vi "PutSpectralData.vi"(0 "shot":i32, 1 "wavelengths":dbl[](array[numeric]), 2 "Counts":dbl[][](array[numeric]), 3 "time":dbl[](array[numeric]), 4 "Integration Times":i32[](array[numeric]), 5 "LensFiber":string, 6 "Radius 1":dbl, 7 "Radius 2":dbl, 8 "Z 1":dbl=-1.0, 9 "Z 2":dbl=1.0, 10 "Angle 1":dbl=157.5, 11 "Angle 2":dbl=157.5, 12 "Comments":string, 13 "backup_directory":path) -> ()   [LabVIEW 2011]
panel:
  in  "Comments Node":string="\\machine::top.usb650:comments"
  in  "LensFiber Node":string="\\machine::top.usb650:setup:su_ft"
  in  "Angle 2 Node":string="\\machine::top.usb650:setup:su_phi2"
  in  "Z 2 Node":string="\\machine::top.usb650:setup:su_z2"
  in  "R 2 Node":string="\\machine::top.usb650:setup:su_maj_r2"
  in  "Angle 1 Node":string="\\machine::top.usb650:setup:su_phi1"
  in  "Z 1 Node":string="\\machine::top.usb650:setup:su_z1"
  in  "R 1 Node":string="\\machine::top.usb650:setup:su_maj_r1"
  in  "Frame Time Node":string="\\machine::top.usb650:framing:frm_start"
  in  "Wavelengths Node":string="\\machine::top.usb650:calib:wve_spec"
  in  "Number of Pixels Node":string="\\machine::top.usb650:setup:su_pixels"
  in  "Number of Frames Node":string="\\machine::top.usb650:framing:frm_n"
  in  "Frame Integration Time Node":string="\\machine::top.usb650:framing:frm_int"
  in  "Frame Counts Node":string="\\machine::top.usb650:raw_spectra"
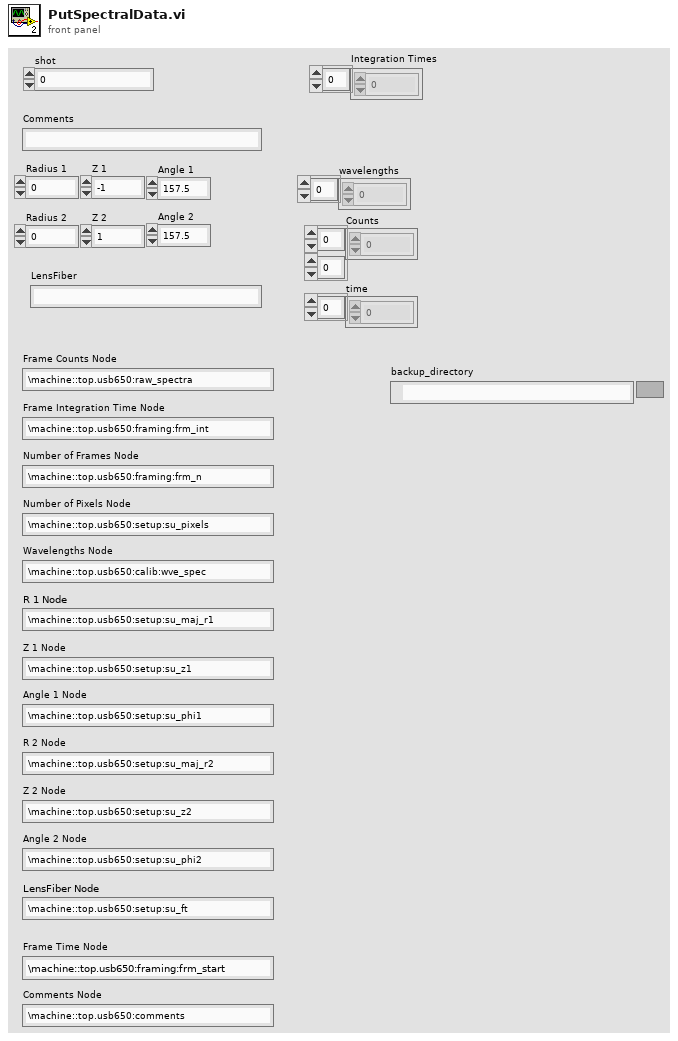
[diagram p1: front panel]
types:
  T1 = enum16{"open", "replace", "create", "open or create", "replace or create", "replace or create with confirmation"}
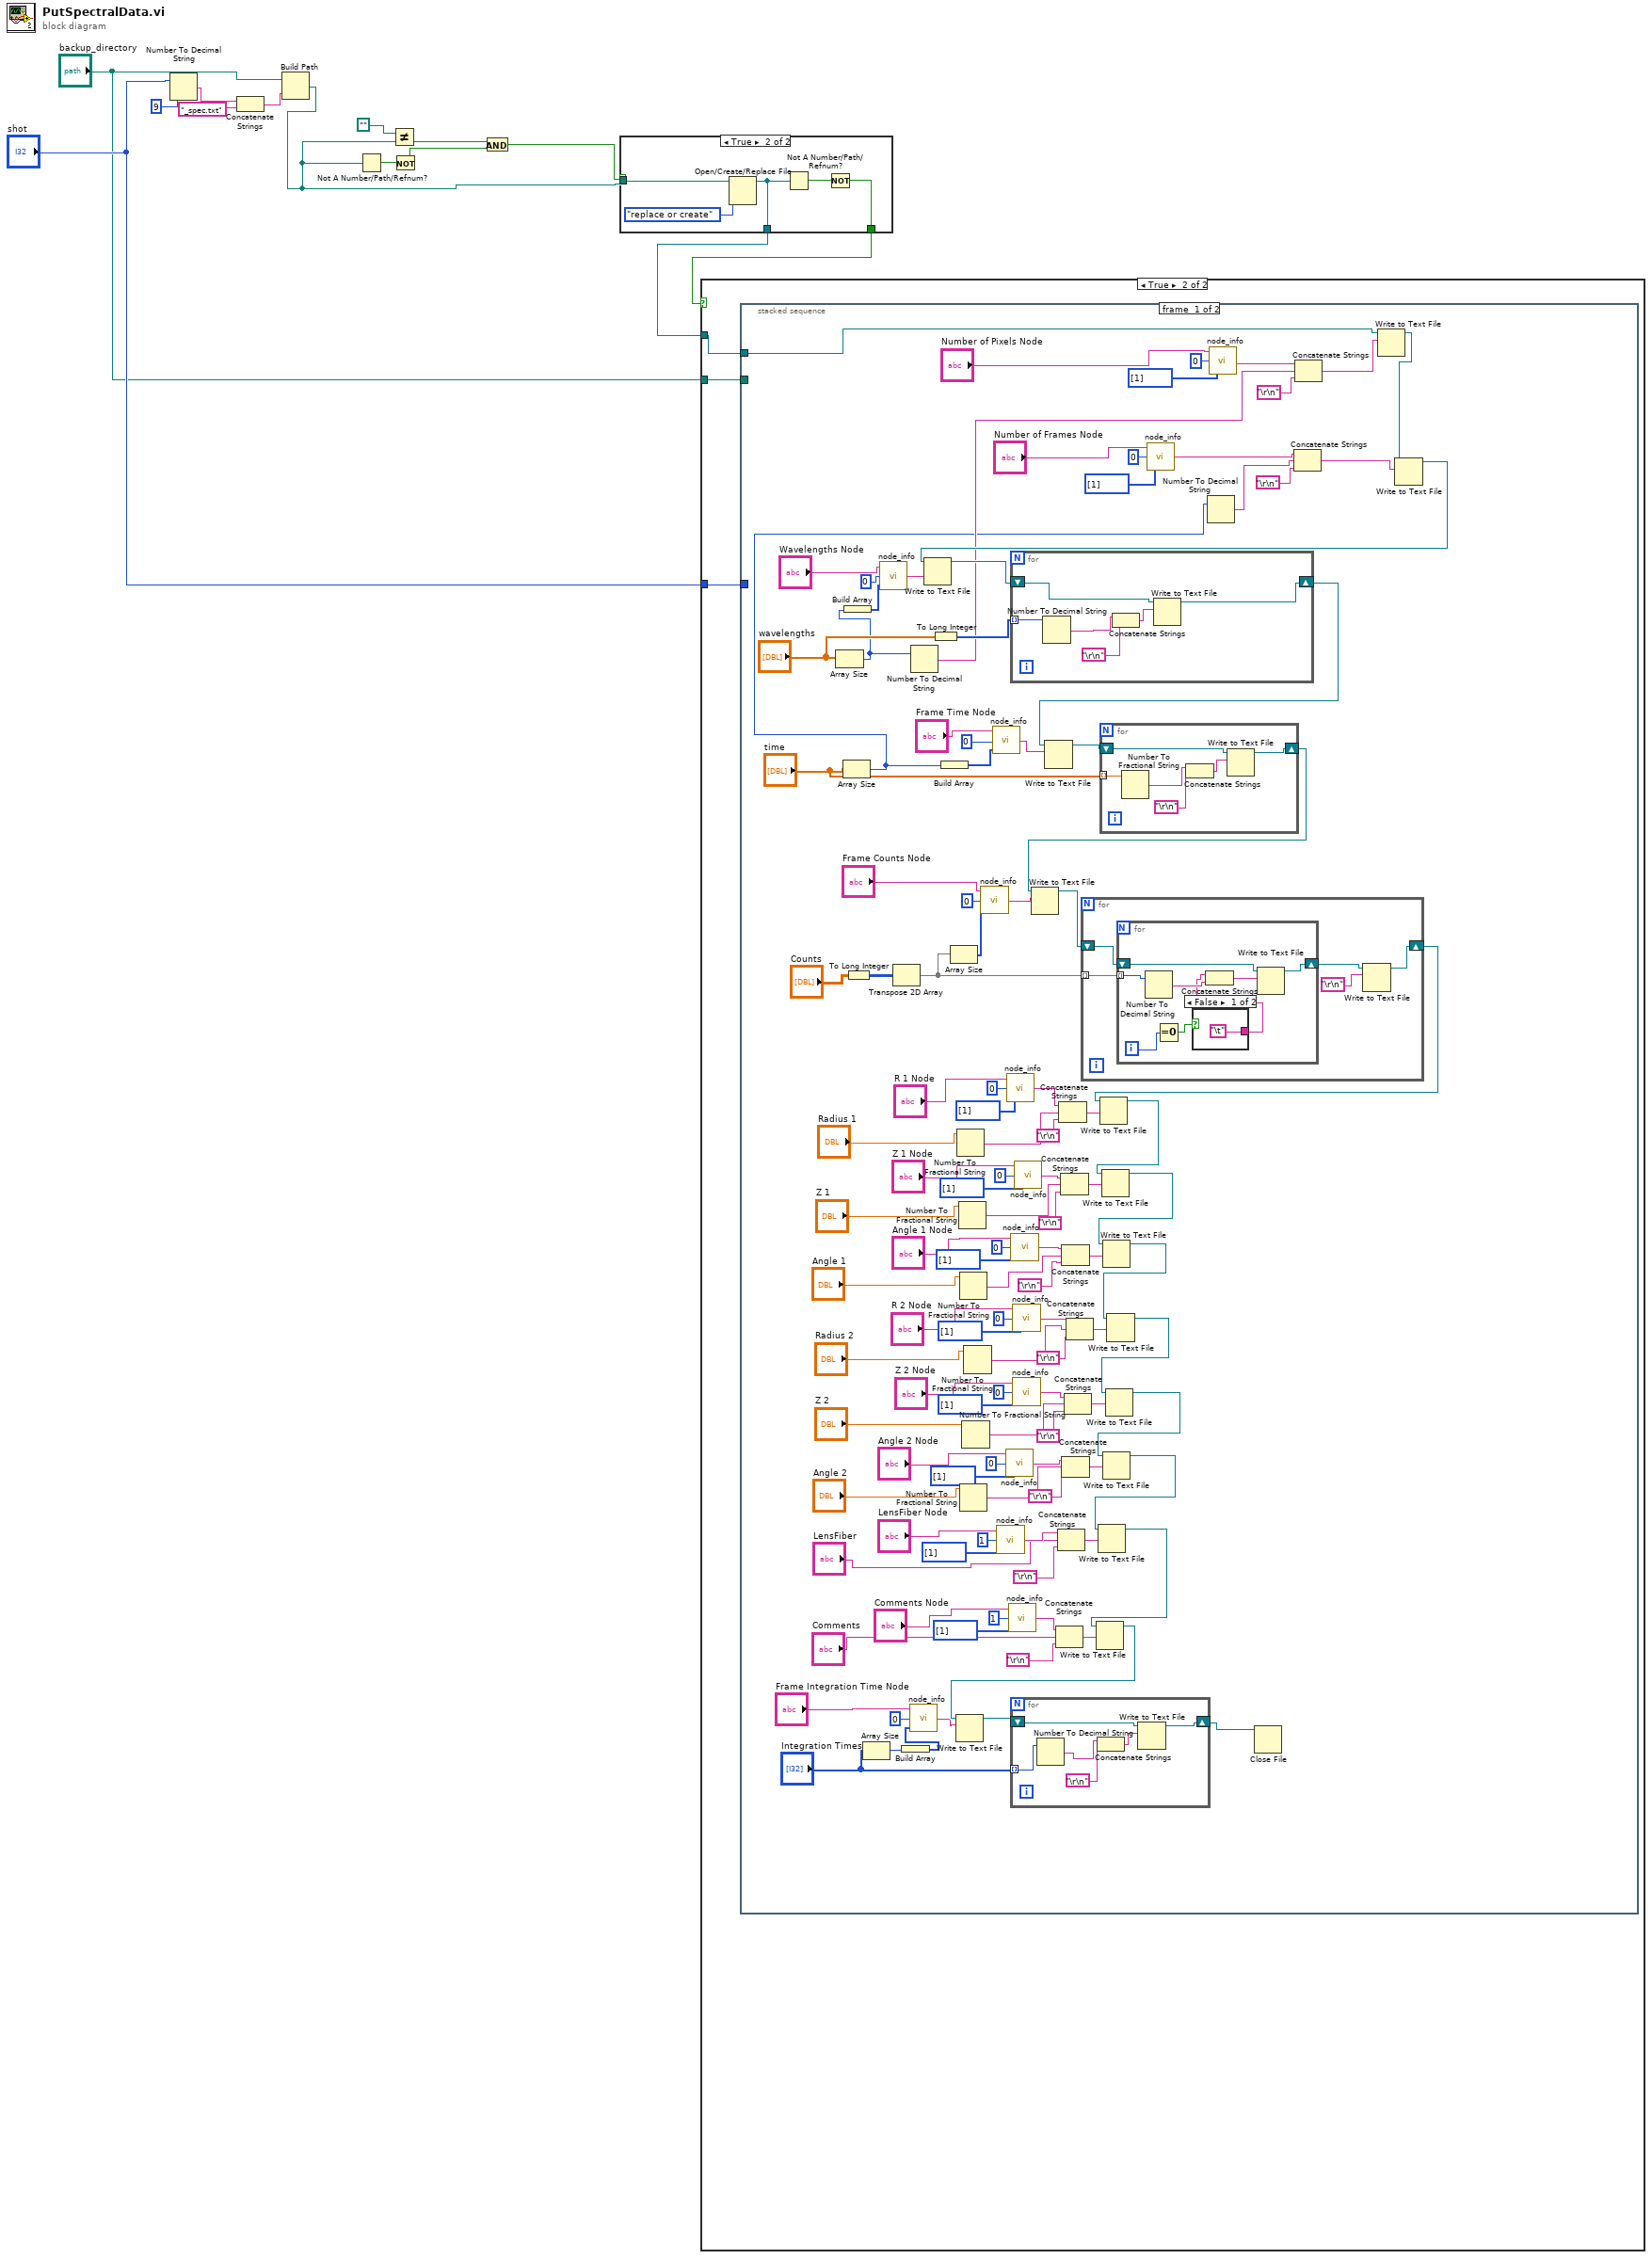
[diagram p0: block diagram]
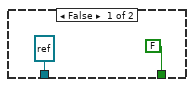
[diagram p2: hidden frame]
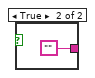
[diagram p4: hidden frame]
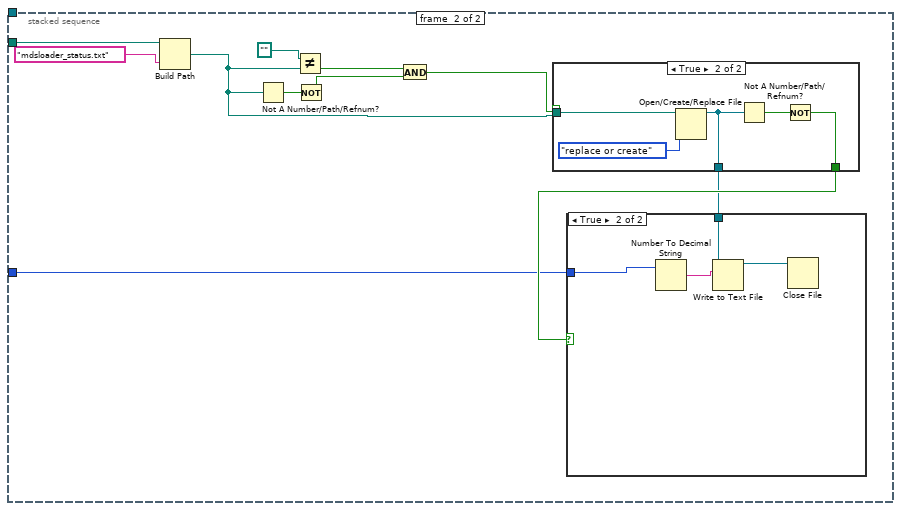
[diagram p5: hidden frame]
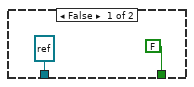
[diagram p7: hidden frame]
diagram:
  n1 = Number To Decimal String(number="shot", width (-)=i16 9) -> (decimal integer string=w5:string)
  n2 = Concatenate Strings(w5, "_spec.txt" ("string")) -> (w6:string)
  n3 = Build Path(base path="backup_directory", name or relative path=w6) -> (appended path=w3:path)
  n4 = Not A Number/Path/Refnum?(number/path/refnum=w3) -> (NaN/Path/Refnum?=w13:bool)
  n5 = Not Equal?(x=path "", y=w3) -> (x != y?=w11:bool)
  n6 = Not(x=w13) -> (.not. x?=w10:bool)
  n7 = And(x=w11, y=w10) -> (x .and. y?=w9:bool)
  n8 = case shown="True" w9 {
    tunnel: [FALSE w19] -> w8
    tunnel: [refnum<file> refnum ("refnum out") w18] -> w14
    tunnel: w3 -> [_ w17]
    frame False {
    }
    frame True {
      n9 = Open/Create/Replace File(file path (use dialog)=w17, operation (0:open)=T1."replace or create") -> (refnum out=w18:refnum<file>)  [unwired: 4 in, 2 out]
      n10 = Not A Number/Path/Refnum?(number/path/refnum=w18) -> (NaN/Path/Refnum?=w20:bool)
      n11 = Not(x=w20) -> (.not. x?=w19:bool)
    }
  }
  n12 = case shown="True" w8 {
    tunnel: w14 -> [_ w24]
    tunnel: "shot" -> [_ w23]
    tunnel: "backup_directory" -> [_ w22]
    frame False {
    }
    frame True {
      n13 = stacked-sequence {
        tunnel: w24 -> [w145 _]
        tunnel: w23 -> [_ w183]
        tunnel: w22 -> [_ w181]
        frame #0 {
          n14 = Array Size(array="wavelengths") -> (size(s)=w93:i32)
          n15 = Array Size(array="time") -> (size(s)=w88:i32)
          n16 = Build Array(w93) -> (w92:i32[])
          n17 = To Long Integer(number="Counts") -> (32bit integer=w86:i32[][])
          n18 = Array Size(array="Integration Times") -> (size(s)=w28:i32)
          n19 = call "node_info.vi"("Length"=w92, "Type"=0, "Name"="Wavelengths Node") -> ("Info"=w26:string)
          n20 = Transpose 2D Array(2D array=w86) -> (transposed array=w85:i32[][])
          n21 = Build Array(w28) -> (w27:i32[])
          n22 = call "node_info.vi"("Length"=w27, "Type"=0, "Name"="Frame Integration Time Node") -> ("Info"=w30:string)
          n23 = Number To Decimal String(number=w93) -> (decimal integer string=w103:string)  [unwired: 1 in]
          n24 = To Long Integer(number="wavelengths") -> (32bit integer=w110:i32[])
          n25 = Build Array(w88) -> (w89:i32[])
          n26 = Array Size(array=w85) -> (size(s)=w83:i32[])
          n27 = Number To Fractional String(number="Radius 1") -> (F-format string=w76:string)  [unwired: 3 in]
          n28 = Number To Fractional String(number="Z 1") -> (F-format string=w72:string)  [unwired: 3 in]
          n29 = Number To Fractional String(number="Angle 1") -> (F-format string=w64:string)  [unwired: 3 in]
          n30 = Number To Fractional String(number="Angle 2") -> (F-format string=w46:string)  [unwired: 3 in]
          n31 = Number To Fractional String(number="Z 2") -> (F-format string=w52:string)  [unwired: 3 in]
          n32 = Number To Fractional String(number="Radius 2") -> (F-format string=w58:string)  [unwired: 3 in]
          n33 = call "node_info.vi"("Length"=w83, "Type"=0, "Name"="Frame Counts Node") -> ("Info"=w84:string)
          n34 = call "node_info.vi"("Length"=w89, "Type"=0, "Name"="Frame Time Node") -> ("Info"=w87:string)
          n35 = call "node_info.vi"("Length"=i32[] [1], "Type"=1, "Name"="LensFiber Node") -> ("Info"=w41:string)
          n36 = call "node_info.vi"("Length"=i32[] [1], "Type"=0, "Name"="Angle 2 Node") -> ("Info"=w47:string)
          n37 = call "node_info.vi"("Length"=i32[] [1], "Type"=0, "Name"="R 1 Node") -> ("Info"=w77:string)
          n38 = call "node_info.vi"("Length"=i32[] [1], "Type"=1, "Name"="Comments Node") -> ("Info"=w35:string)
          n39 = call "node_info.vi"("Length"=i32[] [1], "Type"=0, "Name"="Angle 1 Node") -> ("Info"=w65:string)
          n40 = call "node_info.vi"("Length"=i32[] [1], "Type"=0, "Name"="R 2 Node") -> ("Info"=w59:string)
          n41 = call "node_info.vi"("Length"=i32[] [1], "Type"=0, "Name"="Z 2 Node") -> ("Info"=w53:string)
          n42 = call "node_info.vi"("Length"=i32[] [1], "Type"=0, "Name"="Z 1 Node") -> ("Info"=w73:string)
          n43 = Concatenate Strings(w35, "Comments", "\r\n") -> (w134:string)
          n44 = Concatenate Strings(w41, "LensFiber", "\r\n") -> (w135:string)
          n45 = Concatenate Strings(w77, w76, "\r\n") -> (w141:string)
          n46 = Concatenate Strings(w73, w72, "\r\n") -> (w140:string)
          n47 = Concatenate Strings(w65, w64, "\r\n") -> (w139:string)
          n48 = Concatenate Strings(w47, w46, "\r\n") -> (w136:string)
          n49 = Concatenate Strings(w53, w52, "\r\n") -> (w137:string)
          n50 = Concatenate Strings(w59, w58, "\r\n") -> (w138:string)
          n51 = call "node_info.vi"("Length"=i32[] [1], "Type"=0, "Name"="Number of Frames Node") -> ("Info"=w97:string)
          n52 = Number To Decimal String(number=w88) -> (decimal integer string=w98:string)  [unwired: 1 in]
          n53 = call "node_info.vi"("Length"=i32[] [1], "Type"=0, "Name"="Number of Pixels Node") -> ("Info"=w105:string)
          n54 = Concatenate Strings(w97, w98, "\r\n") -> (w96:string)
          n55 = Concatenate Strings(w105, w103, "\r\n") -> (w25:string)
          n56 = Write to Text File(file (use dialog)=w145, text=w25) -> (refnum out=w144:refnum<file>)  [unwired: 2 in, 2 out]
          n57 = Write to Text File(file (use dialog)=w144, text=w96) -> (refnum out=w121:refnum<file>)  [unwired: 2 in, 2 out]
          n58 = Write to Text File(file (use dialog)=w121, text=w26) -> (refnum out=w143:refnum<file>)  [unwired: 2 in, 2 out]
          n59 = for {
            shift-right: [w176] -> w122
            shift-left: w143 -> [w177]
            tunnel: w110 -> [w174] mode=indexing
            n60 = Number To Decimal String(number=w174) -> (decimal integer string=w173:string)  [unwired: 1 in]
            n61 = Concatenate Strings(w173, "\r\n") -> (w178:string)
            n62 = Write to Text File(file (use dialog)=w177, text=w178) -> (refnum out=w176:refnum<file>)  [unwired: 2 in, 2 out]
          }
          n63 = Write to Text File(file (use dialog)=w122, text=w87) -> (refnum out=w142:refnum<file>)  [unwired: 2 in, 2 out]
          n64 = for {
            shift-right: [w171] -> w120
            shift-left: w142 -> [w170]
            tunnel: "time" -> [w167] mode=indexing
            n65 = Number To Fractional String(number=w167) -> (F-format string=w169:string)  [unwired: 3 in]
            n66 = Concatenate Strings(w169, "\r\n") -> (w172:string)
            n67 = Write to Text File(file (use dialog)=w170, text=w172) -> (refnum out=w171:refnum<file>)  [unwired: 2 in, 2 out]
          }
          n68 = Write to Text File(file (use dialog)=w120, text=w84) -> (refnum out=w119:refnum<file>)  [unwired: 2 in, 2 out]
          n69 = for {
            shift-right: [w147] -> w111
            shift-left: w119 -> [w150]
            tunnel: w85 -> [w149] mode=indexing
            n70 = for {
              shift-right: [w156] -> w148
              shift-left: w150 -> [w157]
              tunnel: w149 -> [w155] mode=indexing
              i -> [w152]
              n71 = Number To Decimal String(number=w155) -> (decimal integer string=w154:string)  [unwired: 1 in]
              n72 = Equal To 0?(x=w152) -> (x = 0?=w153:bool)
              n73 = case shown="False" w153 {
                tunnel: ["\t" ""] -> w151
                frame False {
                }
                frame True {
                }
              }
              n74 = Concatenate Strings(w151, w154) -> (w158:string)
              n75 = Write to Text File(file (use dialog)=w157, text=w158) -> (refnum out=w156:refnum<file>)  [unwired: 2 in, 2 out]
            }
            n76 = Write to Text File(file (use dialog)=w148, text="\r\n") -> (refnum out=w147:refnum<file>)  [unwired: 2 in, 2 out]
          }
          n77 = Write to Text File(file (use dialog)=w111, text=w141) -> (refnum out=w133:refnum<file>)  [unwired: 2 in, 2 out]
          n78 = Write to Text File(file (use dialog)=w133, text=w140) -> (refnum out=w132:refnum<file>)  [unwired: 2 in, 2 out]
          n79 = Write to Text File(file (use dialog)=w132, text=w139) -> (refnum out=w131:refnum<file>)  [unwired: 2 in, 2 out]
          n80 = Write to Text File(file (use dialog)=w131, text=w138) -> (refnum out=w130:refnum<file>)  [unwired: 2 in, 2 out]
          n81 = Write to Text File(file (use dialog)=w130, text=w137) -> (refnum out=w129:refnum<file>)  [unwired: 2 in, 2 out]
          n82 = Write to Text File(file (use dialog)=w129, text=w136) -> (refnum out=w128:refnum<file>)  [unwired: 2 in, 2 out]
          n83 = Write to Text File(file (use dialog)=w128, text=w135) -> (refnum out=w127:refnum<file>)  [unwired: 2 in, 2 out]
          n84 = Write to Text File(file (use dialog)=w127, text=w134) -> (refnum out=w124:refnum<file>)  [unwired: 2 in, 2 out]
          n85 = Write to Text File(file (use dialog)=w124, text=w30) -> (refnum out=w126:refnum<file>)  [unwired: 2 in, 2 out]
          n86 = for {
            shift-right: [w165] -> w125
            shift-left: w126 -> [w164]
            tunnel: "Integration Times" -> [w161] mode=indexing
            n87 = Number To Decimal String(number=w161) -> (decimal integer string=w162:string)  [unwired: 1 in]
            n88 = Concatenate Strings(w162, "\r\n") -> (w166:string)
            n89 = Write to Text File(file (use dialog)=w164, text=w166) -> (refnum out=w165:refnum<file>)  [unwired: 2 in, 2 out]
          }
          n90 = Close File(refnum=w125) -> ()  [unwired: 1 in, 2 out]
        }
        frame #1 {
          n91 = Build Path(base path=w181, name or relative path="mdsloader_status.txt") -> (appended path=w179:path)
          n92 = Not A Number/Path/Refnum?(number/path/refnum=w179) -> (NaN/Path/Refnum?=w189:bool)
          n93 = Not Equal?(x=path "", y=w179) -> (x != y?=w188:bool)
          n94 = Not(x=w189) -> (.not. x?=w187:bool)
          n95 = And(x=w188, y=w187) -> (x .and. y?=w186:bool)
          n96 = case shown="True" w186 {
            tunnel: [FALSE w198] -> w185
            tunnel: [refnum<file> refnum ("refnum out") w197] -> w184
            tunnel: w179 -> [_ w196]
            frame False {
            }
            frame True {
              n97 = Open/Create/Replace File(file path (use dialog)=w196, operation (0:open)=T1."replace or create") -> (refnum out=w197:refnum<file>)  [unwired: 4 in, 2 out]
              n98 = Not A Number/Path/Refnum?(number/path/refnum=w197) -> (NaN/Path/Refnum?=w199:bool)
              n99 = Not(x=w199) -> (.not. x?=w198:bool)
            }
          }
          n100 = case shown="True" w185 {
            tunnel: w184 -> [_ w193]
            tunnel: w183 -> [_ w190]
            frame False {
            }
            frame True {
              n101 = Number To Decimal String(number=w190) -> (decimal integer string=w191:string)  [unwired: 1 in]
              n102 = Write to Text File(file (use dialog)=w193, text=w191) -> (refnum out=w192:refnum<file>)  [unwired: 2 in, 2 out]
              n103 = Close File(refnum=w192) -> ()  [unwired: 1 in, 2 out]
            }
          }
        }
      }
    }
  }
